vi "displayWarnings.vi"(10 "viewThisComponent":refnum<class "ViewThisComponent.lvclass">) -> ()   [LabVIEW 2016, in "EXAViewElements.lvlib"]
doc: "Displays warning information."
uses:
  EXAViewElements.lvlib
  Typedefs/StateValue.ctl
  Typedefs/EXATypedefs.lvlib
  ComponentTemplateCore/ComponentModel/ComponentModel/View/View.lvclass
  ViewThisComponent/ViewThisComponent.lvclass
  home/andres/ct_cmpuserevents/ComponentTemplateCore/ComponentModel/ComponentModel/View/View.lvclass
panel:
  out "LoopTime":dbl[unit] caption="ms"
  out "LoopTimeOutOfRange":bool caption="Loop Time Out Of Range"
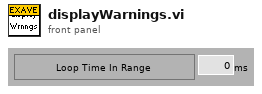
[diagram p1: front panel]
types:
  T1 = typedef "EXATypedefs.lvlib/PubDataEvents.ctl" = cluster{"AppliedSettingsMatchStart":refnum<user-event>, "SettingVersions":refnum<user-event>, "SummaryState":refnum<user-event>, "RejectedCommand":refnum<user-event>, "DetailedState":refnum<user-event>, "ErrorCode":refnum<user-event>, "Heartbeat":refnum<user-event>, "LoopTime_ms":refnum<user-event>, "LoopTimeOutOfRange":refnum<user-event>, "Timestamp":refnum<user-event>}
  T2 = typedef "EXATypedefs.lvlib/StateValue.ctl" = enum16{"", " DisabledState", "EnabledState", "FaultState", "OfflineState", "StandbyState"}
  T3 = enum16{"", " DisabledState", "EnabledState", "FaultState", "OfflineState", "StandbyState"}
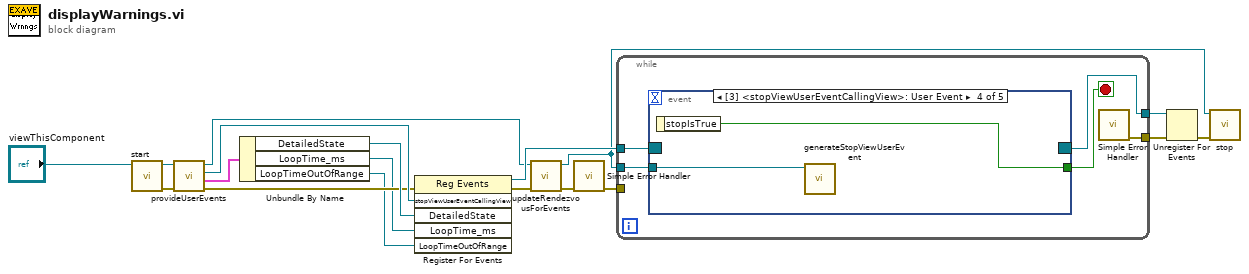
[diagram p0: block diagram]
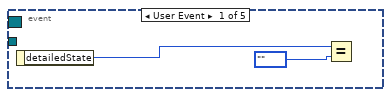
[diagram p2: hidden frame]
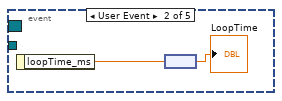
[diagram p3: hidden frame]
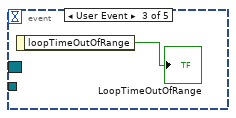
[diagram p4: hidden frame]
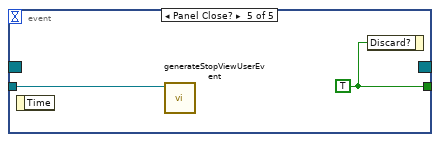
[diagram p5: hidden frame]
diagram:
  n1 = call-dynamic "start.vi"("View in"="viewThisComponent") -> ("error out"=w13:errorcluster, "View out"=w14:refnum<class "ViewThisComponent.lvclass">)  [unwired: 9 in]
  n2 = call "provideUserEvents.vi"("error in (no error)"=w13, "ViewThisComponent in"=w14) -> ("error out"=w12:errorcluster, "pubDataEvents"=w15:T1, "stopViewUserEventCallingView"=w16:refnum<user-event>, "ViewThisComponent out"=w2:refnum<class "ViewThisComponent.lvclass">)  [unwired: 6 in]
  n3 = Unbundle By Name(w15) -> ("DetailedState"=w17:refnum<user-event>, "LoopTime_ms"=w9:refnum<user-event>, "LoopTimeOutOfRange"=w8:refnum<user-event>)
  n4 = register-events(error in=w12, w16, w17, w9, w8) -> (reference out=w7:refnum<event-registration>, error out=w4:errorcluster)  [unwired: 1 in]
  n5 = call "updateRendezvousForEvents.vi"("error in (no error)"=w4, "View in"=w2) -> ("error out"=w3:errorcluster, "View out"=w1:refnum<class "ViewThisComponent.lvclass">)  [unwired: 8 in]
  n6 = call <vilib>:"Simple Error Handler.vi"("error in (no error)"=w3) -> ("error out"=w5:errorcluster)  [unwired: 4 in, 4 out]
  n7 = while {
    tunnel: w7 -> [w23]
    tunnel: w1 -> [w22]
    tunnel: [w20] -> w11
    tunnel: [w19] -> w6
    tunnel: w5 -> [_]
    stop <- w21 stop-if-true
    n8 = event shown="[3] <stopViewUserEventCallingView>: User Event" {
      selector: w23 -> [_ _ _ _ _]
      dyn-events: [_ _ _ _ _] -> w20
      timeout: _ -> [_ _ _ _ _]
      tunnel: w22 -> [_ _ _ w30 w32]
      tunnel: [_ _ _ w29 w31] -> w21
      event User Event {
        n9 = event-data() -> ("detailedState"=w25:T3)  [unwired: 1 in]
        n10 = Equal?(x=w25, y=StateValue."" ("StateValue")) -> ()  [unwired: 1 out]
      }
      event User Event {
        n11 = event-data() -> ("loopTime_ms"=w26:dbl)  [unwired: 1 in]
        n12 = node(w26) -> (→"LoopTime":dbl[unit])
      }
      event User Event {
        n13 = event-data() -> ("loopTimeOutOfRange"=→"LoopTimeOutOfRange":bool)  [unwired: 1 in]
      }
      event User Event {
        n14 = event-data() -> ("stopIsTrue"=w29:bool)  [unwired: 1 in]
        n15 = call "generateStopViewUserEvent.vi"("View in"=w30) -> ()  [unwired: 9 in, 2 out]
      }
      event Panel Close? {
        w31 = TRUE ("Discard?")
        n16 = event-data() -> ()  [unwired: 1 in, 1 out]
        n17 = call "generateStopViewUserEvent.vi"("View in"=w32) -> ()  [unwired: 9 in, 2 out]
        n18 = event-data("Discard?"=w31) -> ()  [unwired: 1 in, 1 out]
      }
    }
    n19 = call <vilib>:"Simple Error Handler.vi"() -> ("error out"=w19:errorcluster)  [unwired: 5 in, 4 out]
  }
  n20 = Unregister For Events(event registration refnum=w11, error in=w6) -> (error out=w10:errorcluster)
  n21 = call-dynamic "stop.vi"("error in (no error)"=w10, "View in"=w1) -> ()  [unwired: 8 in, 2 out]
